vi "filter_strain_9237_test.vi"() -> ()   [LabVIEW 2014]
uses:
  <vilib>/rvi/Analysis/host/Butterworth/config/Butterworth Filter Order.ctl
  <vilib>/rvi/Analysis/host/Butterworth/config/Butterworth Filter Type.ctl
  <vilib>/FPGAPlugInAG/cRIO-9039/niLvFpga_Open_cRIO-9039.vi
  <vilib>/rvi/interface/common/dynamic/niFpgaDynamicAddResources.vi
  <vilib>/rvi/Analysis/host/Butterworth/config/BwScaledCoefficients.vi
  <vilib>/Utility/error.llb/Error Cluster From Error Code.vi
  <vilib>/rvi/errors/niLvFpgaAdjustHostInterfaceError.vi
  <vilib>/FPGAPlugInAG/Dynamic/niLvFpga_Close_Dynamic.vi
  <vilib>/rvi/interface/nirviOpenFPGA/nirviOpenFPGA.xnode
  FPGA Bitfiles/test0304_FPGATarget_strain9237filter_WXVzv8KXAvg.lvbitx
  Yu-Shen/force_control_lys/FPGA VIs/sub VIs/strain_9237_filter_test.vi
  <vilib>/rvi/Analysis/host/Butterworth/XNode/ButterworthCoefficients.xnode
  <vilib>/rvi/interface/nirviReadWriteControl/nirviReadWriteControl.xnode
  <vilib>/rvi/interface/nirviCloseFPGA/nirviCloseFPGA.xnode
  NiFpgaLv.dll
  <vilib>/rvi/interface/Simulation/niFpgaSimulationCallBeginRW.vi
  <vilib>/rvi/Analysis/host/Public/NI_FpgaMspHost.lvlib
panel:
  in  "stop":bool
  in  "sr_p Avg2 (S/s)":dbl=50000.0
  in  "sr_p Avg4 (S/s)":dbl=50000.0
  in  "sr_p Avg8 (S/s)":dbl=50000.0
  in  "fcu_p Avg2 (Hz)":dbl=1000.0
  in  "fcu_p Avg4 (Hz)":dbl=1000.0
  in  "fcu_p Avg8 (Hz)":dbl=1000.0
  in  "sr_p w. f (S/s)":dbl=50000.0
  in  "fcu_p w. f (Hz)":dbl=1000.0
  in  "sr_y Avg2 (S/s)":dbl=50000.0
  in  "fcu_y Avg2 (Hz)":dbl=1000.0
  in  "sr_y Avg4 (S/s)":dbl=50000.0
  in  "fcu_y Avg4 (Hz)":dbl=1000.0
  in  "sr_y Avg8 (S/s)":dbl=50000.0
  in  "fcu_y Avg8 (Hz)":dbl=1000.0
  in  "sr_y w. f (S/s)":dbl=50000.0
  in  "fcu_y w. f (Hz)":dbl=1000.0
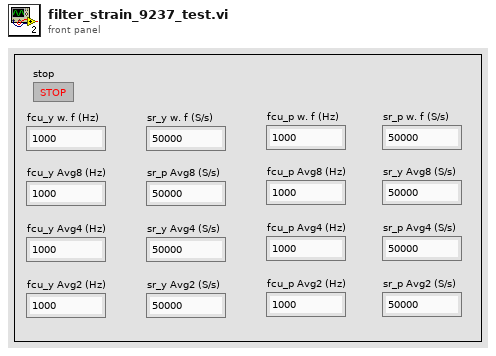
[diagram p1: front panel]
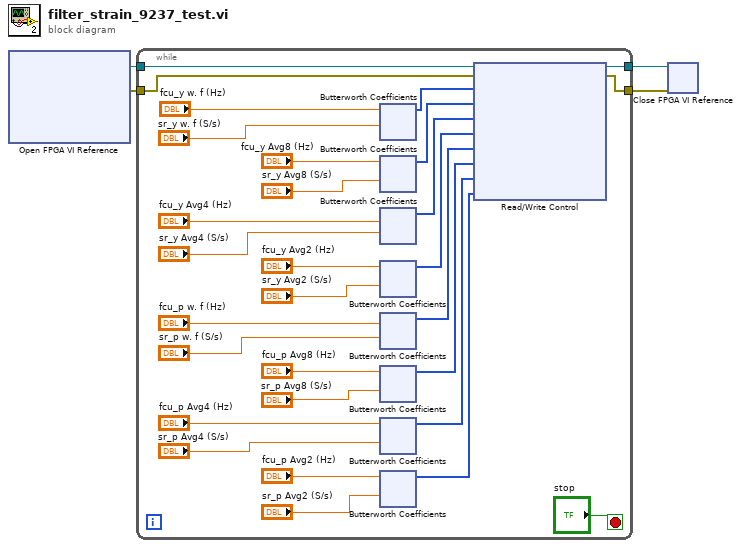
[diagram p0: block diagram]
diagram:
  n1 = xnode "Open FPGA VI Reference"() -> ("FPGA VI Reference Out"=w4:refnum<k20>, "error out"=w1:errorcluster)  [unwired: 2 in]
  n2 = while {
    tunnel: [w31] -> w3
    tunnel: w4 -> [w30]
    tunnel: [w33] -> w2
    tunnel: w1 -> [w32]
    stop <- "stop" stop-if-true
    n3 = xnode "Butterworth Coefficients"("cutoff frequency (Hz)"="fcu_y w. f (Hz)", "sample rate (S/s)"="sr_y w. f (S/s)") -> ("scaled coefficients"=w29:i32[])  [unwired: 1 in, 1 out]
    n4 = xnode "Butterworth Coefficients"("cutoff frequency (Hz)"="fcu_y Avg8 (Hz)", "sample rate (S/s)"="sr_y Avg8 (S/s)") -> ("scaled coefficients"=w28:i32[])  [unwired: 1 in, 1 out]
    n5 = xnode "Butterworth Coefficients"("cutoff frequency (Hz)"="fcu_y Avg4 (Hz)", "sample rate (S/s)"="sr_y Avg4 (S/s)") -> ("scaled coefficients"=w27:i32[])  [unwired: 1 in, 1 out]
    n6 = xnode "Butterworth Coefficients"("cutoff frequency (Hz)"="fcu_y Avg2 (Hz)", "sample rate (S/s)"="sr_y Avg2 (S/s)") -> ("scaled coefficients"=w26:i32[])  [unwired: 1 in, 1 out]
    n7 = xnode "Butterworth Coefficients"("cutoff frequency (Hz)"="fcu_p w. f (Hz)", "sample rate (S/s)"="sr_p w. f (S/s)") -> ("scaled coefficients"=w25:i32[])  [unwired: 1 in, 1 out]
    n8 = xnode "Butterworth Coefficients"("cutoff frequency (Hz)"="fcu_p Avg8 (Hz)", "sample rate (S/s)"="sr_p Avg8 (S/s)") -> ("scaled coefficients"=w24:i32[])  [unwired: 1 in, 1 out]
    n9 = xnode "Butterworth Coefficients"("cutoff frequency (Hz)"="fcu_p Avg4 (Hz)", "sample rate (S/s)"="sr_p Avg4 (S/s)") -> ("scaled coefficients"=w23:i32[])  [unwired: 1 in, 1 out]
    n10 = xnode "Butterworth Coefficients"("cutoff frequency (Hz)"="fcu_p Avg2 (Hz)", "sample rate (S/s)"="sr_p Avg2 (S/s)") -> ("scaled coefficients"=w22:i32[])  [unwired: 1 in, 1 out]
    n11 = xnode "Read/Write Control"("FPGA VI Reference In"=w30, "error in"=w32, "Strain_y coefficients"=w29, "Strain_y_Avg8 coeff."=w28, "Strain_y_Avg4 coeff."=w27, "Strain_y_Avg2 coeff."=w26, "Strain_p coefficients"=w25, "Strain_p_Avg8 coeff."=w24, "Strain_p_Avg4 coeff."=w23, "Strain_p_Avg2 coeff."=w22) -> ("FPGA VI Reference Out"=w31:refnum<k20>, "error out"=w33:errorcluster)
  }
  n12 = xnode "Close FPGA VI Reference"("FPGA VI Reference In"=w3, "error in"=w2) -> ()  [unwired: 1 out]
